vi "AddMeasurement.vi"(7 "measurement_group id":u16, 8 "error in (no error)":errorcluster, 9 "misura_strumento":sgl, 10 "misura_riferimento":sgl, 11 "ByteGSAPIBase in":refnum<class "ByteGSAPIBase.lvclass">) -> (0 "error out":errorcluster, 2 "Measurement data":T1, 3 "ByteGSAPIBase out":refnum<class "ByteGSAPIBase.lvclass">)   [LabVIEW 2019, in "ByteGSWebAPI.lvlib" / "ByteGSAPIBase.lvclass"]
uses:
  ByteGSAPIBase.lvclass
  MeasurementResData.ctl
  <vilib>/Bytelabs/ByteREST/ByteRESTClass/ByteRESTBase/HTTP/Status_Code.ctl
  AddMeasurementReqData.ctl
  ByteGSAPIBase.lvclass/ByteGSAPIBase.ctl
  <vilib>/Bytelabs/ByteREST/ByteRESTClass/ByteRESTBase/RESTBase.lvclass
  <vilib>/numeric/Random Number (Range) U64.vi
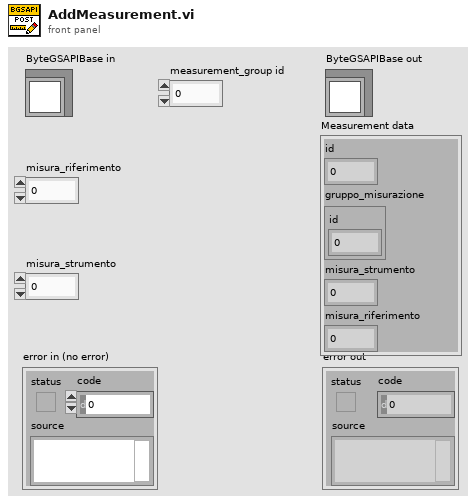
[diagram p1: front panel]
types:
  T1 = typedef "ByteGSWebAPI.lvlib/ByteGSAPIBase.lvclass/MeasurementResData.ctl" = cluster{"id":i32, "gruppo_misurazione":cluster{"id":i32}, "misura_strumento":dbl, "misura_riferimento":dbl}
  T2 = typedef "ByteGSWebAPI.lvlib/ByteGSAPIBase.lvclass/AddMeasurementReqData.ctl" = cluster{"misura_strumento":sgl, "misura_riferimento":sgl, "gruppo_misurazione":cluster{"id":i32}}
  T3 = typedef "ByteREST.lvlib/RESTBase.lvclass/Status_Code.ctl" = u16
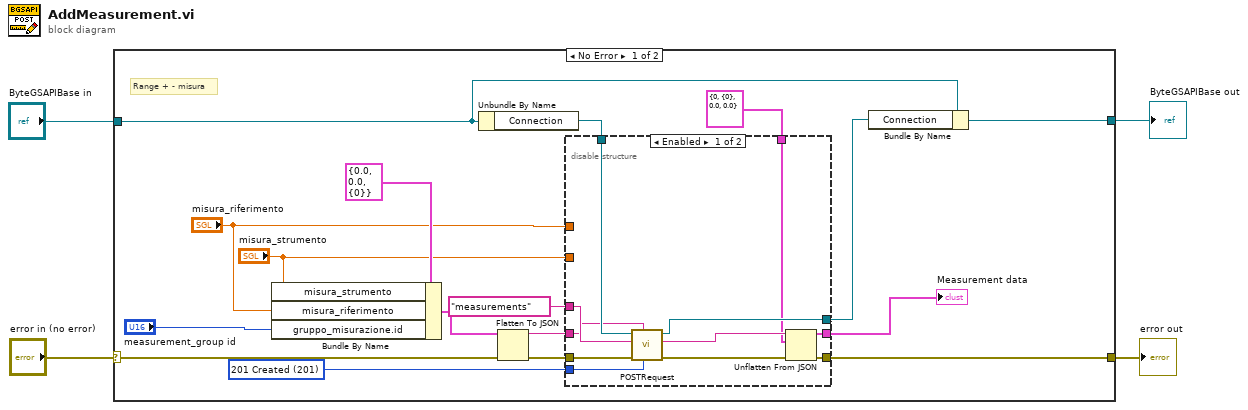
[diagram p0: block diagram]
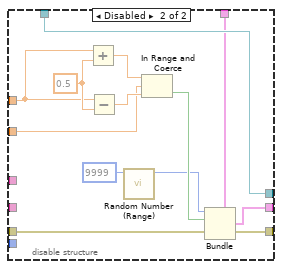
[diagram p2: hidden frame]
diagram:
  n1 = case shown="No Error" "error in (no error)" {
    selector: "error in (no error)" -> [w14 w46]
    tunnel: [w8 w46] -> w3
    tunnel: [w19 w45] -> w1
    tunnel: "ByteGSAPIBase in" -> [w21 w45]
    frame No Error {
      w16 = T3 201 items=["200 OK"=200, "201 Created"=201, "400 Bad Request"=400, "401 Unauthorized"=401, "403 Forbidden"=403, "404 Not Found"=404, "405 Method Not Allowed"=405, "406 Not Acceptable"=406, "500 Internal Server Error"=500] ("expected response")
      # "Range + - misura"
      n2 = Bundle By Name(cluster=T2 {"misura_strumento"=0.0, "misura_riferimento"=0.0, "gruppo_misurazione"={"id"=0}} ("Valori"), "misura_strumento"="misura_strumento", "misura_riferimento"="misura_riferimento", "gruppo_misurazione.id"="measurement_group id") -> (w12:T2)
      n3 = Unbundle By Name(w21) -> ("Connection"=w20:refnum<class "RESTBase.lvclass">)
      n4 = Flatten To JSON(anything=w12, error in (no error)=w14) -> (JSON string=w10:string, 11:w13:errorcluster)  [unwired: 1 in]
      n5 = disable-structure shown="Enabled" {
        disable-tunnel: w20 -> [w32 w37]
        disable-tunnel: [w31 w37] -> w18
        disable-tunnel: "measurements" ("Request") -> [w30 _]
        disable-tunnel: w16 -> [w29 _]
        disable-tunnel: w13 -> [w28 w33]
        disable-tunnel: w10 -> [w27 _]
        disable-tunnel: T1 {"id"=0, "gruppo_misurazione"={"id"=0}, "misura_strumento"=0.0, "misura_riferimento"=0.0} -> [w24 w35]
        disable-tunnel: [w23 w39] -> w5
        disable-tunnel: [w22 w33] -> w8
        disable-tunnel: "misura_riferimento" -> [_ w40]
        disable-tunnel: "misura_strumento" -> [_ w41]
        frame Enabled {
          n6 = call-dynamic "POSTRequest.vi"("expected response"=w29, "Body in"=w27, "error in (no error)"=w28, "Request"=w30, "ByteRESTBase in"=w32) -> ("error out"=w25:errorcluster, "Body"=w26:string, "ByteRESTBase out"=w31:refnum<class "RESTBase.lvclass">)  [unwired: 3 in, 1 out]
          n7 = Unflatten From JSON(JSON string=w26, type and defaults=w24, error in (no error)=w25) -> (value=w23:T1, error out=w22:errorcluster)  [unwired: 4 in]
        }
        frame Disabled {
          w42 = 0.5
          n8 = Add(x=w40, y=w42) -> (x+y=w43:dbl)
          n9 = Subtract(x=w40, y=w42) -> (x-y=w44:dbl)
          n10 = call-poly <vilib>:"Random Number (Range).vi"("upper bound (100)"=u64 9999) -> ("number"=w34:u64)  [unwired: 10 in]
          n11 = In Range and Coerce(upper limit=w43, x=w41, lower limit=w44) -> (In Range?=w38:bool)  [unwired: 1 out]
          n12 = Bundle(cluster=w35, "id"=w34, "gruppo_misurazione"=w38) -> (w39:T1)  [unwired: 2 in]
        }
      }
      "Measurement data" <- w5
      n13 = Bundle By Name(cluster=w21, "Connection"=w18) -> (w19:refnum<class "ByteGSAPIBase.lvclass">)
    }
    frame Error {
    }
  }
  "error out" <- w3
  "ByteGSAPIBase out" <- w1
